vi "CalcRobotsVel.vi"(10 "fps":dbl=120.0 format="%#_13g", 11 "Array of robots":T1[](array[typedef]) {"height" format="%+4.3f"; "pixel_y" format="%+4.3f"; "pixel_x" format="%+4.3f"; "orientation" format="%+4.3f"; "y" format="%+4.3f"; "confidence" format="%4.3f"; "x" format="%+4.3f"}) -> (3 "Array of robots":T1[](array[typedef]) {"height" format="%+4.3f"; "pixel_y" format="%+4.3f"; "pixel_x" format="%+4.3f"; "orientation" format="%+4.3f"; "y" format="%+4.3f"; "confidence" format="%4.3f"; "x" format="%+4.3f"})   [LabVIEW 2018]
uses:
  Old vision/Controls/SSL Detection Robot.ctl
  <vilib>/Analysis/Matrix/Datatypes/RealMatrix.ctl
  Utilities_class/Utilities.lvclass
  <vilib>/Analysis/Matrix/NI_Matrix.lvlib
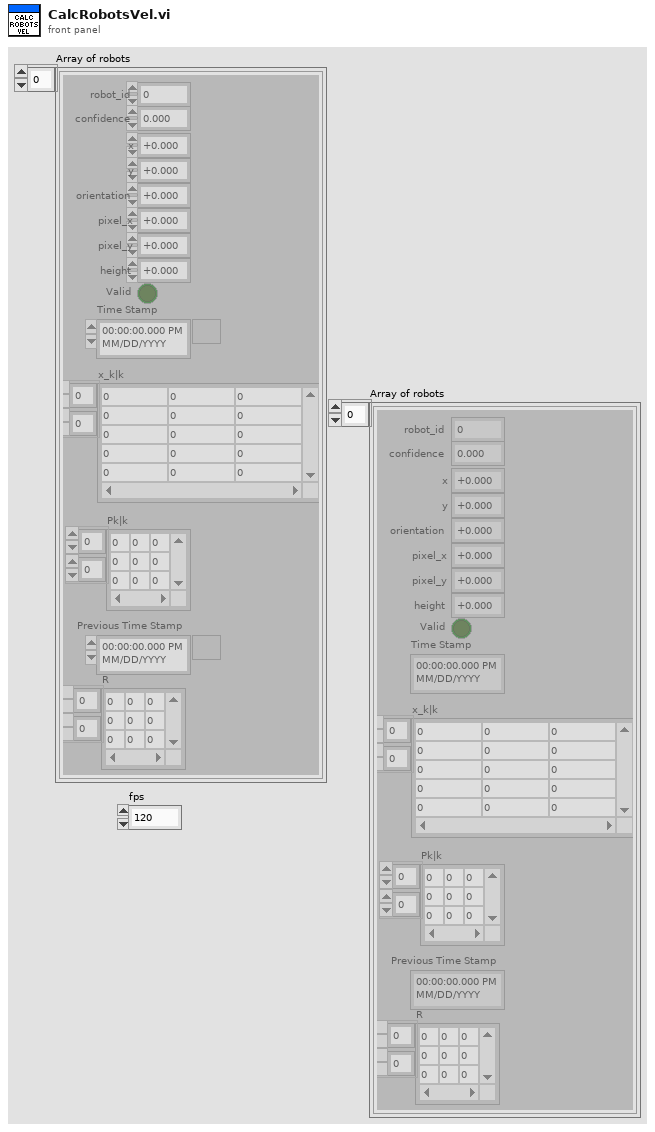
[diagram p1: front panel]
types:
  T1 = typedef "SSL Detection Robot.ctl" = cluster{"x":sgl, "robot_id":u32, "confidence":sgl, "y":sgl, "orientation":sgl, "pixel_x":sgl, "pixel_y":sgl, "height":sgl, "Valid":bool, "Time Stamp":timestamp, "x_k|k":T2, "Pk|k":T2, "Previous Time Stamp":timestamp, "R":T2}
  T2 = typedef "NI_Matrix.lvlib/RealMatrix.ctl" = dbl[][]
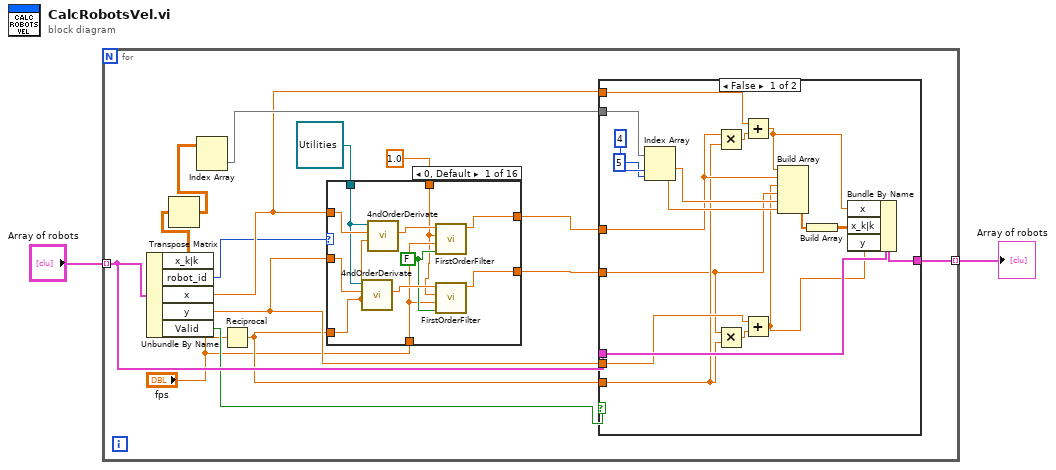
[diagram p0: block diagram]
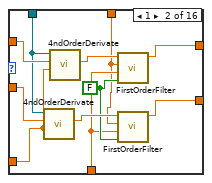
[diagram p2: hidden frame]
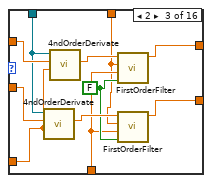
[diagram p3: hidden frame]
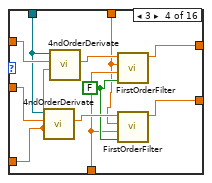
[diagram p4: hidden frame]
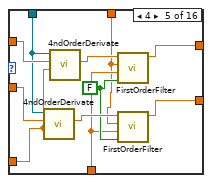
[diagram p5: hidden frame]
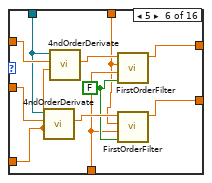
[diagram p6: hidden frame]
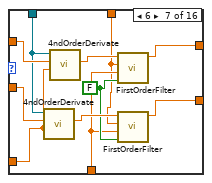
[diagram p7: hidden frame]
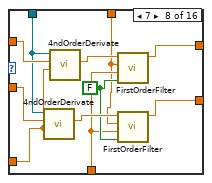
[diagram p8: hidden frame]
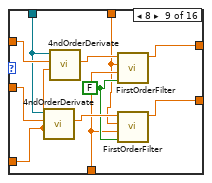
[diagram p9: hidden frame]
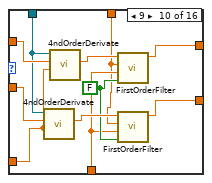
[diagram p10: hidden frame]
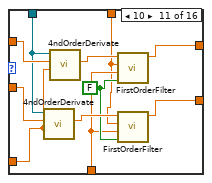
[diagram p11: hidden frame]
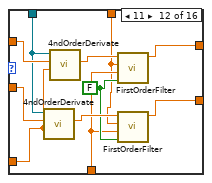
[diagram p12: hidden frame]
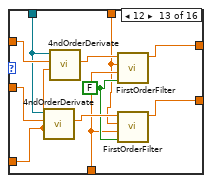
[diagram p13: hidden frame]
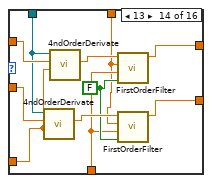
[diagram p14: hidden frame]
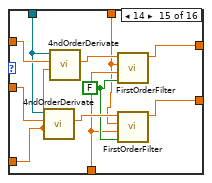
[diagram p15: hidden frame]
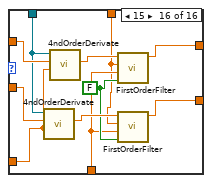
[diagram p16: hidden frame]
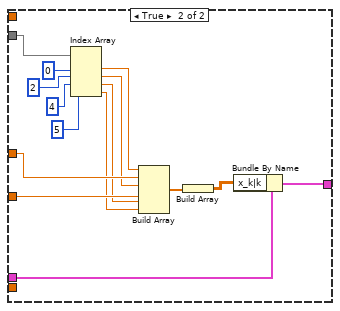
[diagram p17: hidden frame]
diagram:
  n1 = for {
    tunnel: "Array of robots" -> [w17] mode=indexing
    tunnel: [w16] -> w1 mode=indexing
    n2 = Unbundle By Name(w17) -> ("x_k|k"=w8:T2, "robot_id"=w6:u32, "x"=w14:sgl, "y"=w12:sgl, "Valid"=w9:bool)
    n3 = Transpose Matrix(1:w8) -> (0:w7:T2)
    n4 = Index Array(array=w7) -> (element=w15:dbl[])  [unwired: 2 in]
    n5 = Reciprocal(x="fps") -> (1/x=w11:dbl)
    n6 = case shown="0, Default" w6 {
      tunnel: w14 -> [w28 w39 w50 w61 w72 w83 w94 w105 w116 w127 w138 w149 w160 w171 w182 w193]
      tunnel: [w26 w37 w48 w59 w70 w81 w92 w103 w114 w125 w136 w147 w158 w169 w180 w191] -> w13
      tunnel: w12 -> [w20 w31 w42 w53 w64 w75 w86 w97 w108 w119 w130 w141 w152 w163 w174 w185]
      tunnel: w11 -> [w18 w29 w40 w51 w62 w73 w84 w95 w106 w117 w128 w139 w150 w161 w172 w183]
      tunnel: [w21 w32 w43 w54 w65 w76 w87 w98 w109 w120 w131 w142 w153 w164 w175 w186] -> w10
      tunnel: refnum<class "Utilities.lvclass"> refnum ("Utilities in") -> [w19 w30 w41 w52 w63 w74 w85 w96 w107 w118 w129 w140 w151 w162 w173 w184]
      tunnel: 1.0 -> [w22 w33 w44 w55 w66 w77 w88 w99 w110 w121 w132 w143 w154 w165 w176 w187]
      tunnel: "fps" -> [w23 w34 w45 w56 w67 w78 w89 w100 w111 w122 w133 w144 w155 w166 w177 w188]
      frame 0, Default {
        w24 = FALSE
        n7 = call "4ndOrderDerivate.vi"("dt"=w18, "x"=w20, "Utilities in"=w19) -> ("dx/dt"=w25:dbl)  [unwired: 6 in, 2 out]
        n8 = call "4ndOrderDerivate.vi"("dt"=w18, "x"=w28, "Utilities in"=w19) -> ("dx/dt"=w27:dbl)  [unwired: 6 in, 2 out]
        n9 = call "FirstOrderFilter.vi"("ball?"=w24, "fps"=w23, "fc"=w22, "Numeric in"=w27) -> ("Numeric out"=w26:dbl)  [unwired: 7 in]
        n10 = call "FirstOrderFilter.vi"("ball?"=w24, "fps"=w23, "fc"=w22, "Numeric in"=w25) -> ("Numeric out"=w21:dbl)  [unwired: 7 in]
      }
      frame 1 {
        w35 = FALSE
        n11 = call "4ndOrderDerivate.vi"("dt"=w29, "x"=w31, "Utilities in"=w30) -> ("dx/dt"=w36:dbl)  [unwired: 6 in, 2 out]
        n12 = call "4ndOrderDerivate.vi"("dt"=w29, "x"=w39, "Utilities in"=w30) -> ("dx/dt"=w38:dbl)  [unwired: 6 in, 2 out]
        n13 = call "FirstOrderFilter.vi"("ball?"=w35, "fps"=w34, "fc"=w33, "Numeric in"=w38) -> ("Numeric out"=w37:dbl)  [unwired: 7 in]
        n14 = call "FirstOrderFilter.vi"("ball?"=w35, "fps"=w34, "fc"=w33, "Numeric in"=w36) -> ("Numeric out"=w32:dbl)  [unwired: 7 in]
      }
      frame 2 {
        w46 = FALSE
        n15 = call "4ndOrderDerivate.vi"("dt"=w40, "x"=w42, "Utilities in"=w41) -> ("dx/dt"=w47:dbl)  [unwired: 6 in, 2 out]
        n16 = call "4ndOrderDerivate.vi"("dt"=w40, "x"=w50, "Utilities in"=w41) -> ("dx/dt"=w49:dbl)  [unwired: 6 in, 2 out]
        n17 = call "FirstOrderFilter.vi"("ball?"=w46, "fps"=w45, "fc"=w44, "Numeric in"=w49) -> ("Numeric out"=w48:dbl)  [unwired: 7 in]
        n18 = call "FirstOrderFilter.vi"("ball?"=w46, "fps"=w45, "fc"=w44, "Numeric in"=w47) -> ("Numeric out"=w43:dbl)  [unwired: 7 in]
      }
      frame 3 {
        w57 = FALSE
        n19 = call "4ndOrderDerivate.vi"("dt"=w51, "x"=w53, "Utilities in"=w52) -> ("dx/dt"=w58:dbl)  [unwired: 6 in, 2 out]
        n20 = call "4ndOrderDerivate.vi"("dt"=w51, "x"=w61, "Utilities in"=w52) -> ("dx/dt"=w60:dbl)  [unwired: 6 in, 2 out]
        n21 = call "FirstOrderFilter.vi"("ball?"=w57, "fps"=w56, "fc"=w55, "Numeric in"=w60) -> ("Numeric out"=w59:dbl)  [unwired: 7 in]
        n22 = call "FirstOrderFilter.vi"("ball?"=w57, "fps"=w56, "fc"=w55, "Numeric in"=w58) -> ("Numeric out"=w54:dbl)  [unwired: 7 in]
      }
      frame 4 {
        w68 = FALSE
        n23 = call "4ndOrderDerivate.vi"("dt"=w62, "x"=w64, "Utilities in"=w63) -> ("dx/dt"=w69:dbl)  [unwired: 6 in, 2 out]
        n24 = call "4ndOrderDerivate.vi"("dt"=w62, "x"=w72, "Utilities in"=w63) -> ("dx/dt"=w71:dbl)  [unwired: 6 in, 2 out]
        n25 = call "FirstOrderFilter.vi"("ball?"=w68, "fps"=w67, "fc"=w66, "Numeric in"=w71) -> ("Numeric out"=w70:dbl)  [unwired: 7 in]
        n26 = call "FirstOrderFilter.vi"("ball?"=w68, "fps"=w67, "fc"=w66, "Numeric in"=w69) -> ("Numeric out"=w65:dbl)  [unwired: 7 in]
      }
      frame 5 {
        w79 = FALSE
        n27 = call "4ndOrderDerivate.vi"("dt"=w73, "x"=w75, "Utilities in"=w74) -> ("dx/dt"=w80:dbl)  [unwired: 6 in, 2 out]
        n28 = call "4ndOrderDerivate.vi"("dt"=w73, "x"=w83, "Utilities in"=w74) -> ("dx/dt"=w82:dbl)  [unwired: 6 in, 2 out]
        n29 = call "FirstOrderFilter.vi"("ball?"=w79, "fps"=w78, "fc"=w77, "Numeric in"=w82) -> ("Numeric out"=w81:dbl)  [unwired: 7 in]
        n30 = call "FirstOrderFilter.vi"("ball?"=w79, "fps"=w78, "fc"=w77, "Numeric in"=w80) -> ("Numeric out"=w76:dbl)  [unwired: 7 in]
      }
      frame 6 {
        w90 = FALSE
        n31 = call "4ndOrderDerivate.vi"("dt"=w84, "x"=w86, "Utilities in"=w85) -> ("dx/dt"=w91:dbl)  [unwired: 6 in, 2 out]
        n32 = call "4ndOrderDerivate.vi"("dt"=w84, "x"=w94, "Utilities in"=w85) -> ("dx/dt"=w93:dbl)  [unwired: 6 in, 2 out]
        n33 = call "FirstOrderFilter.vi"("ball?"=w90, "fps"=w89, "fc"=w88, "Numeric in"=w93) -> ("Numeric out"=w92:dbl)  [unwired: 7 in]
        n34 = call "FirstOrderFilter.vi"("ball?"=w90, "fps"=w89, "fc"=w88, "Numeric in"=w91) -> ("Numeric out"=w87:dbl)  [unwired: 7 in]
      }
      frame 7 {
        w101 = FALSE
        n35 = call "4ndOrderDerivate.vi"("dt"=w95, "x"=w97, "Utilities in"=w96) -> ("dx/dt"=w102:dbl)  [unwired: 6 in, 2 out]
        n36 = call "4ndOrderDerivate.vi"("dt"=w95, "x"=w105, "Utilities in"=w96) -> ("dx/dt"=w104:dbl)  [unwired: 6 in, 2 out]
        n37 = call "FirstOrderFilter.vi"("ball?"=w101, "fps"=w100, "fc"=w99, "Numeric in"=w104) -> ("Numeric out"=w103:dbl)  [unwired: 7 in]
        n38 = call "FirstOrderFilter.vi"("ball?"=w101, "fps"=w100, "fc"=w99, "Numeric in"=w102) -> ("Numeric out"=w98:dbl)  [unwired: 7 in]
      }
      frame 8 {
        w112 = FALSE
        n39 = call "4ndOrderDerivate.vi"("dt"=w106, "x"=w108, "Utilities in"=w107) -> ("dx/dt"=w113:dbl)  [unwired: 6 in, 2 out]
        n40 = call "4ndOrderDerivate.vi"("dt"=w106, "x"=w116, "Utilities in"=w107) -> ("dx/dt"=w115:dbl)  [unwired: 6 in, 2 out]
        n41 = call "FirstOrderFilter.vi"("ball?"=w112, "fps"=w111, "fc"=w110, "Numeric in"=w115) -> ("Numeric out"=w114:dbl)  [unwired: 7 in]
        n42 = call "FirstOrderFilter.vi"("ball?"=w112, "fps"=w111, "fc"=w110, "Numeric in"=w113) -> ("Numeric out"=w109:dbl)  [unwired: 7 in]
      }
      frame 9 {
        w123 = FALSE
        n43 = call "4ndOrderDerivate.vi"("dt"=w117, "x"=w119, "Utilities in"=w118) -> ("dx/dt"=w124:dbl)  [unwired: 6 in, 2 out]
        n44 = call "4ndOrderDerivate.vi"("dt"=w117, "x"=w127, "Utilities in"=w118) -> ("dx/dt"=w126:dbl)  [unwired: 6 in, 2 out]
        n45 = call "FirstOrderFilter.vi"("ball?"=w123, "fps"=w122, "fc"=w121, "Numeric in"=w126) -> ("Numeric out"=w125:dbl)  [unwired: 7 in]
        n46 = call "FirstOrderFilter.vi"("ball?"=w123, "fps"=w122, "fc"=w121, "Numeric in"=w124) -> ("Numeric out"=w120:dbl)  [unwired: 7 in]
      }
      frame 10 {
        w134 = FALSE
        n47 = call "4ndOrderDerivate.vi"("dt"=w128, "x"=w130, "Utilities in"=w129) -> ("dx/dt"=w135:dbl)  [unwired: 6 in, 2 out]
        n48 = call "4ndOrderDerivate.vi"("dt"=w128, "x"=w138, "Utilities in"=w129) -> ("dx/dt"=w137:dbl)  [unwired: 6 in, 2 out]
        n49 = call "FirstOrderFilter.vi"("ball?"=w134, "fps"=w133, "fc"=w132, "Numeric in"=w137) -> ("Numeric out"=w136:dbl)  [unwired: 7 in]
        n50 = call "FirstOrderFilter.vi"("ball?"=w134, "fps"=w133, "fc"=w132, "Numeric in"=w135) -> ("Numeric out"=w131:dbl)  [unwired: 7 in]
      }
      frame 11 {
        w145 = FALSE
        n51 = call "4ndOrderDerivate.vi"("dt"=w139, "x"=w141, "Utilities in"=w140) -> ("dx/dt"=w146:dbl)  [unwired: 6 in, 2 out]
        n52 = call "4ndOrderDerivate.vi"("dt"=w139, "x"=w149, "Utilities in"=w140) -> ("dx/dt"=w148:dbl)  [unwired: 6 in, 2 out]
        n53 = call "FirstOrderFilter.vi"("ball?"=w145, "fps"=w144, "fc"=w143, "Numeric in"=w148) -> ("Numeric out"=w147:dbl)  [unwired: 7 in]
        n54 = call "FirstOrderFilter.vi"("ball?"=w145, "fps"=w144, "fc"=w143, "Numeric in"=w146) -> ("Numeric out"=w142:dbl)  [unwired: 7 in]
      }
      frame 12 {
        w156 = FALSE
        n55 = call "4ndOrderDerivate.vi"("dt"=w150, "x"=w152, "Utilities in"=w151) -> ("dx/dt"=w157:dbl)  [unwired: 6 in, 2 out]
        n56 = call "4ndOrderDerivate.vi"("dt"=w150, "x"=w160, "Utilities in"=w151) -> ("dx/dt"=w159:dbl)  [unwired: 6 in, 2 out]
        n57 = call "FirstOrderFilter.vi"("ball?"=w156, "fps"=w155, "fc"=w154, "Numeric in"=w159) -> ("Numeric out"=w158:dbl)  [unwired: 7 in]
        n58 = call "FirstOrderFilter.vi"("ball?"=w156, "fps"=w155, "fc"=w154, "Numeric in"=w157) -> ("Numeric out"=w153:dbl)  [unwired: 7 in]
      }
      frame 13 {
        w167 = FALSE
        n59 = call "4ndOrderDerivate.vi"("dt"=w161, "x"=w163, "Utilities in"=w162) -> ("dx/dt"=w168:dbl)  [unwired: 6 in, 2 out]
        n60 = call "4ndOrderDerivate.vi"("dt"=w161, "x"=w171, "Utilities in"=w162) -> ("dx/dt"=w170:dbl)  [unwired: 6 in, 2 out]
        n61 = call "FirstOrderFilter.vi"("ball?"=w167, "fps"=w166, "fc"=w165, "Numeric in"=w170) -> ("Numeric out"=w169:dbl)  [unwired: 7 in]
        n62 = call "FirstOrderFilter.vi"("ball?"=w167, "fps"=w166, "fc"=w165, "Numeric in"=w168) -> ("Numeric out"=w164:dbl)  [unwired: 7 in]
      }
      frame 14 {
        w178 = FALSE
        n63 = call "4ndOrderDerivate.vi"("dt"=w172, "x"=w174, "Utilities in"=w173) -> ("dx/dt"=w179:dbl)  [unwired: 6 in, 2 out]
        n64 = call "4ndOrderDerivate.vi"("dt"=w172, "x"=w182, "Utilities in"=w173) -> ("dx/dt"=w181:dbl)  [unwired: 6 in, 2 out]
        n65 = call "FirstOrderFilter.vi"("ball?"=w178, "fps"=w177, "fc"=w176, "Numeric in"=w181) -> ("Numeric out"=w180:dbl)  [unwired: 7 in]
        n66 = call "FirstOrderFilter.vi"("ball?"=w178, "fps"=w177, "fc"=w176, "Numeric in"=w179) -> ("Numeric out"=w175:dbl)  [unwired: 7 in]
      }
      frame 15 {
        w189 = FALSE
        n67 = call "4ndOrderDerivate.vi"("dt"=w183, "x"=w185, "Utilities in"=w184) -> ("dx/dt"=w190:dbl)  [unwired: 6 in, 2 out]
        n68 = call "4ndOrderDerivate.vi"("dt"=w183, "x"=w193, "Utilities in"=w184) -> ("dx/dt"=w192:dbl)  [unwired: 6 in, 2 out]
        n69 = call "FirstOrderFilter.vi"("ball?"=w189, "fps"=w188, "fc"=w187, "Numeric in"=w192) -> ("Numeric out"=w191:dbl)  [unwired: 7 in]
        n70 = call "FirstOrderFilter.vi"("ball?"=w189, "fps"=w188, "fc"=w187, "Numeric in"=w190) -> ("Numeric out"=w186:dbl)  [unwired: 7 in]
      }
    }
    n71 = case shown="False" w9 {
      tunnel: w17 -> [w211 w225]
      tunnel: [w210 w226] -> w16
      tunnel: w15 -> [w208 w223]
      tunnel: w14 -> [w202 _]
      tunnel: w13 -> [w200 w220]
      tunnel: w12 -> [w198 _]
      tunnel: w11 -> [w197 _]
      tunnel: w10 -> [w196 w218]
      frame False {
        n72 = Index Array(array=w208, index #1=4, index #2=5) -> (element #1=w204:dbl, element #2=w203:dbl)
        n73 = Multiply(x=w200, y=w197) -> (x*y=w201:dbl)
        n74 = Multiply(x=w196, y=w197) -> (x*y=w199:dbl)
        n75 = Add(x=w202, y=w201) -> (x+y=w195:dbl)
        n76 = Add(x=w198, y=w199) -> (x+y=w194:dbl)
        n77 = Build Array(w195, w200, w194, w196, w204, w203) -> (w207:dbl[])
        n78 = Build Array(w207) -> (w209:T2)
        n79 = Bundle By Name(cluster=w211, "x"=w195, "x_k|k"=w209, "y"=w194) -> (w210:T1)
      }
      frame True {
        n80 = Index Array(array=w223, index #1=0, index #2=2, index #3=4, index #4=5) -> (element #1=w221:dbl, element #2=w219:dbl, element #3=w217:dbl, element #4=w216:dbl)
        n81 = Build Array(w221, w220, w219, w218, w217, w216) -> (w222:dbl[])
        n82 = Build Array(w222) -> (w224:T2)
        n83 = Bundle By Name(cluster=w225, "x_k|k"=w224) -> (w226:T1)
      }
    }
  }
  "Array of robots" <- w1
